vi "SetTempConfig.vi"(1 "Error In":errorcluster, 2 "Temp Configuration":T1) -> (0 "Error Out":errorcluster)   [LabVIEW 2014]
uses:
  TempConfig.ctl
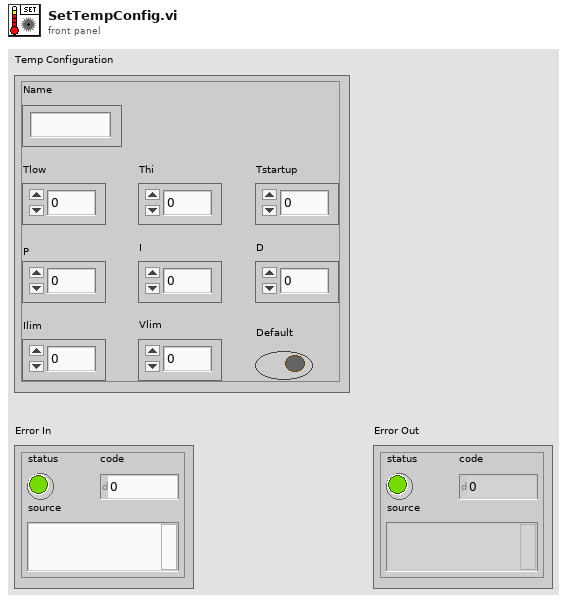
[diagram p1: front panel]
types:
  T1 = typedef "TempConfig.ctl" = cluster{"Name":string, "Thi":dbl, "Tlow":dbl, "Tstartup":dbl, "P":dbl, "I":dbl, "D":dbl, "Ilim":dbl, "Vlim":dbl, "Default":bool}
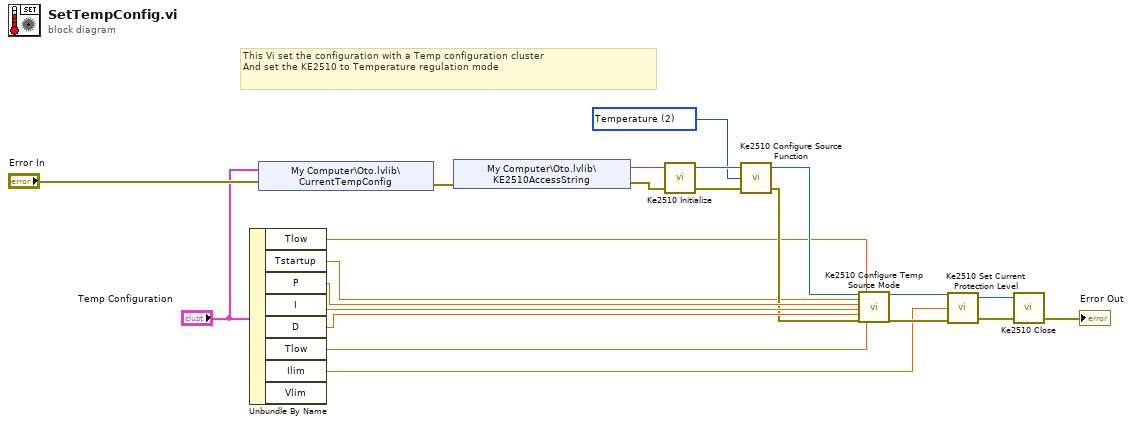
[diagram p0: block diagram]
diagram:
  w16 = 2 items=["Voltage", "Current", "Temperature", "Resistance"] ("function")
  # "This Vi set the configuration with a Temp configuration cluster\nAnd set the KE2510 to Temperature regulation mode"
  n1 = Unbundle By Name("Temp Configuration") -> ("Tlow"=w2:dbl, "Tstartup"=w3:dbl, "P"=w14:dbl, "I"=w13:dbl, "D"=w12:dbl, "Tlow"=w11:dbl, "Ilim"=w7:dbl)  [unwired: 1 out]
  n2 = shared-variable "My Computer\\Oto.lvlib\\CurrentTempConfig"("Temp Configuration", error in="Error In") -> (error out=w20:errorcluster)
  n3 = shared-variable "My Computer\\Oto.lvlib\\KE2510AccessString"(error in=w20) -> (w21:string, error out=w19:errorcluster)
  n4 = call <instrlib>:"Ke2510 Initialize.vi"("error in (no error)"=w19, "resource name"=w21) -> ("error out"=w18:errorcluster, "instrument handle"=w17:refnum<visa-resource-name>)  [unwired: 1 in, 1 out]
  n5 = call <instrlib>:"Ke2510 Configure Source Function.vi"("error in (no error)"=w18, "function"=w16, "instrument handle"=w17) -> ("error out"=w10:errorcluster, "instrument handle out"=w15:refnum<visa-resource-name>)  [unwired: 1 out]
  n6 = call <instrlib>:"Ke2510 Configure Temp Source Mode.vi"("instrument handle"=w15, "setpoint"=w3, "p"=w14, "i"=w13, "d"=w12, "error in (no error)"=w10, "low limit"=w2, "high limit"=w11) -> ("instrument handle out"=w9:refnum<visa-resource-name>, "error out"=w8:errorcluster)  [unwired: 9 in, 1 out]
  n7 = call <instrlib>:"Ke2510 Set Current Protection Level.vi"("error in (no error)"=w8, "value"=w7, "instrument handle"=w9) -> ("error out"=w6:errorcluster, "instrument handle out"=w5:refnum<visa-resource-name>)  [unwired: 1 out]
  n8 = call <instrlib>:"Ke2510 Close.vi"("instrument handle"=w5, "error in (no error)"=w6) -> ("error out"=→"Error Out":errorcluster)  [unwired: 1 in, 1 out]
